vi "Apply DSF Configuration.vi"(8 "error in (no error)":errorcluster, 10 "path":path, 11 "Item Ref in":T1 format="%.0x") -> (0 "error out":errorcluster)   [LabVIEW 2017, in "Data Sharing Framework System Explorer.lvlib"]
uses:
  Data Sharing Framework System Explorer.lvlib
  <vilib>/NI Veristand/Custom Device API/Custom Device Item Ref.ctl
  dsf core/Source/DSF Configuration API/1.0.0/Public/Read All Item IDs/Read All Plugin IDs.vi
  dsf core/Source/DSF Configuration API/1.0.0/DSF Configuration API.lvlib
  <vilib>/NI VeriStand/Custom Device API/Custom Device API.lvlib
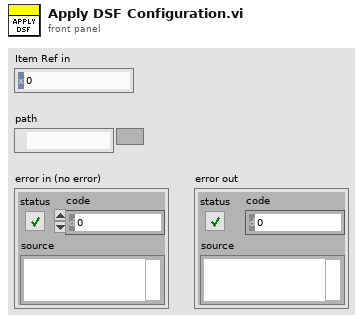
[diagram p1: front panel]
types:
  T1 = typedef "Custom Device API.lvlib/Custom Device Item Ref.ctl" = u64
  T2 = typedef "DSF Configuration API.lvlib/DSF Config Data RefNum.ctl" = refnum<k1>
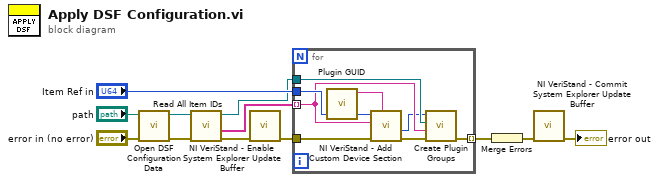
[diagram p0: block diagram]
diagram:
  n1 = call "Open DSF Configuration Data.vi"("error in (no error)"="error in (no error)", "dsf configuration file path"="path") -> ("error out"=w5:errorcluster, "dsf refnum"=w6:T2)  [unwired: 5 in, 3 out]
  n2 = call-poly "Read All Item IDs.vi"("error in (no error)"=w5, "dsf refnum"=w6) -> ("error out"=w2:errorcluster, "Plugin IDs"=w7:string[], "dsf refnum out"=w9:T2)  [unwired: 7 in]
  n3 = call <vilib>:"NI VeriStand - Enable System Explorer Update Buffer.vi"("error in (no error)"=w2) -> ("error out"=w1:errorcluster)  [unwired: 10 in]
  n4 = for {
    tunnel: w7 -> [w15] mode=indexing
    tunnel: "Item Ref in" -> [w20]
    tunnel: w1 -> [w19]
    tunnel: [w16] -> w8 mode=indexing
    tunnel: w9 -> [w18]
    n5 = call "Plugin GUID.vi"() -> ("GUID"=w13:string)  [unwired: 11 in]
    n6 = call <vilib>:"NI VeriStand - Add Custom Device Section.vi"("GUID (Default Section)"=w13, "error in (no error)"=w19, "Section Name"=w15, "Parent Ref in"=w20) -> ("error out"=w17:errorcluster, "Section Ptr"=w14:T1)  [unwired: 4 in, 2 out]
    n7 = call "Create Plugin Groups.vi"("error in (no error)"=w17, "String"=w15, "dsf refnum in"=w18, "Section Ptr"=w14) -> ("error out"=w16:errorcluster)  [unwired: 7 in]
  }
  n8 = Merge Errors(w8) -> (w4:errorcluster)
  n9 = call <vilib>:"NI VeriStand - Commit System Explorer Update Buffer.vi"("error in (no error)"=w4) -> ("error out"=→"error out":errorcluster)  [unwired: 10 in]
